vi "RunFileRenameAddDate.vi"() -> ()   [LabVIEW 2012]
panel:
  out "path out 3":path
  out "filenames 3":string[](array[string])
  out "folder names 3":string[](array[string])
  out "array":string[][](array[string])
  out "filenames":string[](array[string])
  out "folder names":string[](array[string])
  in  "path":path=path "G:/DCIM"
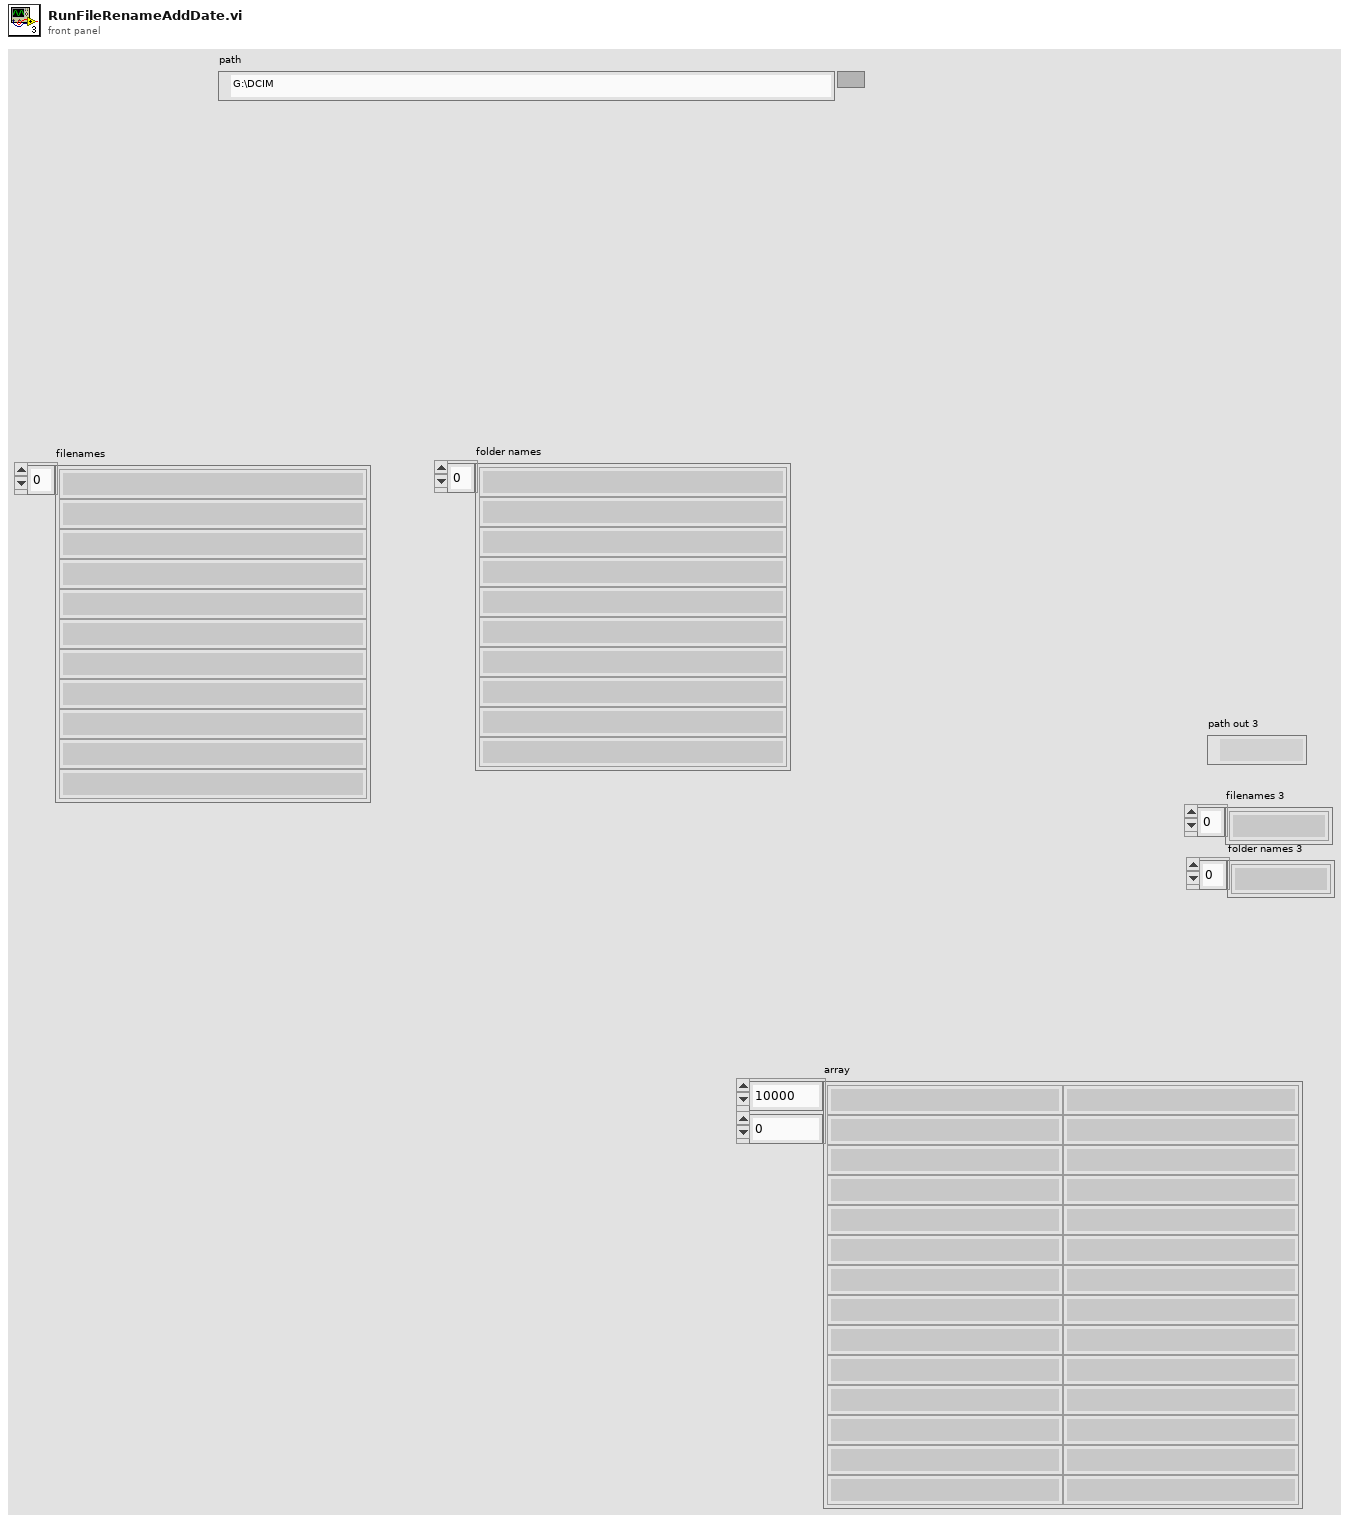
[diagram p1: front panel]
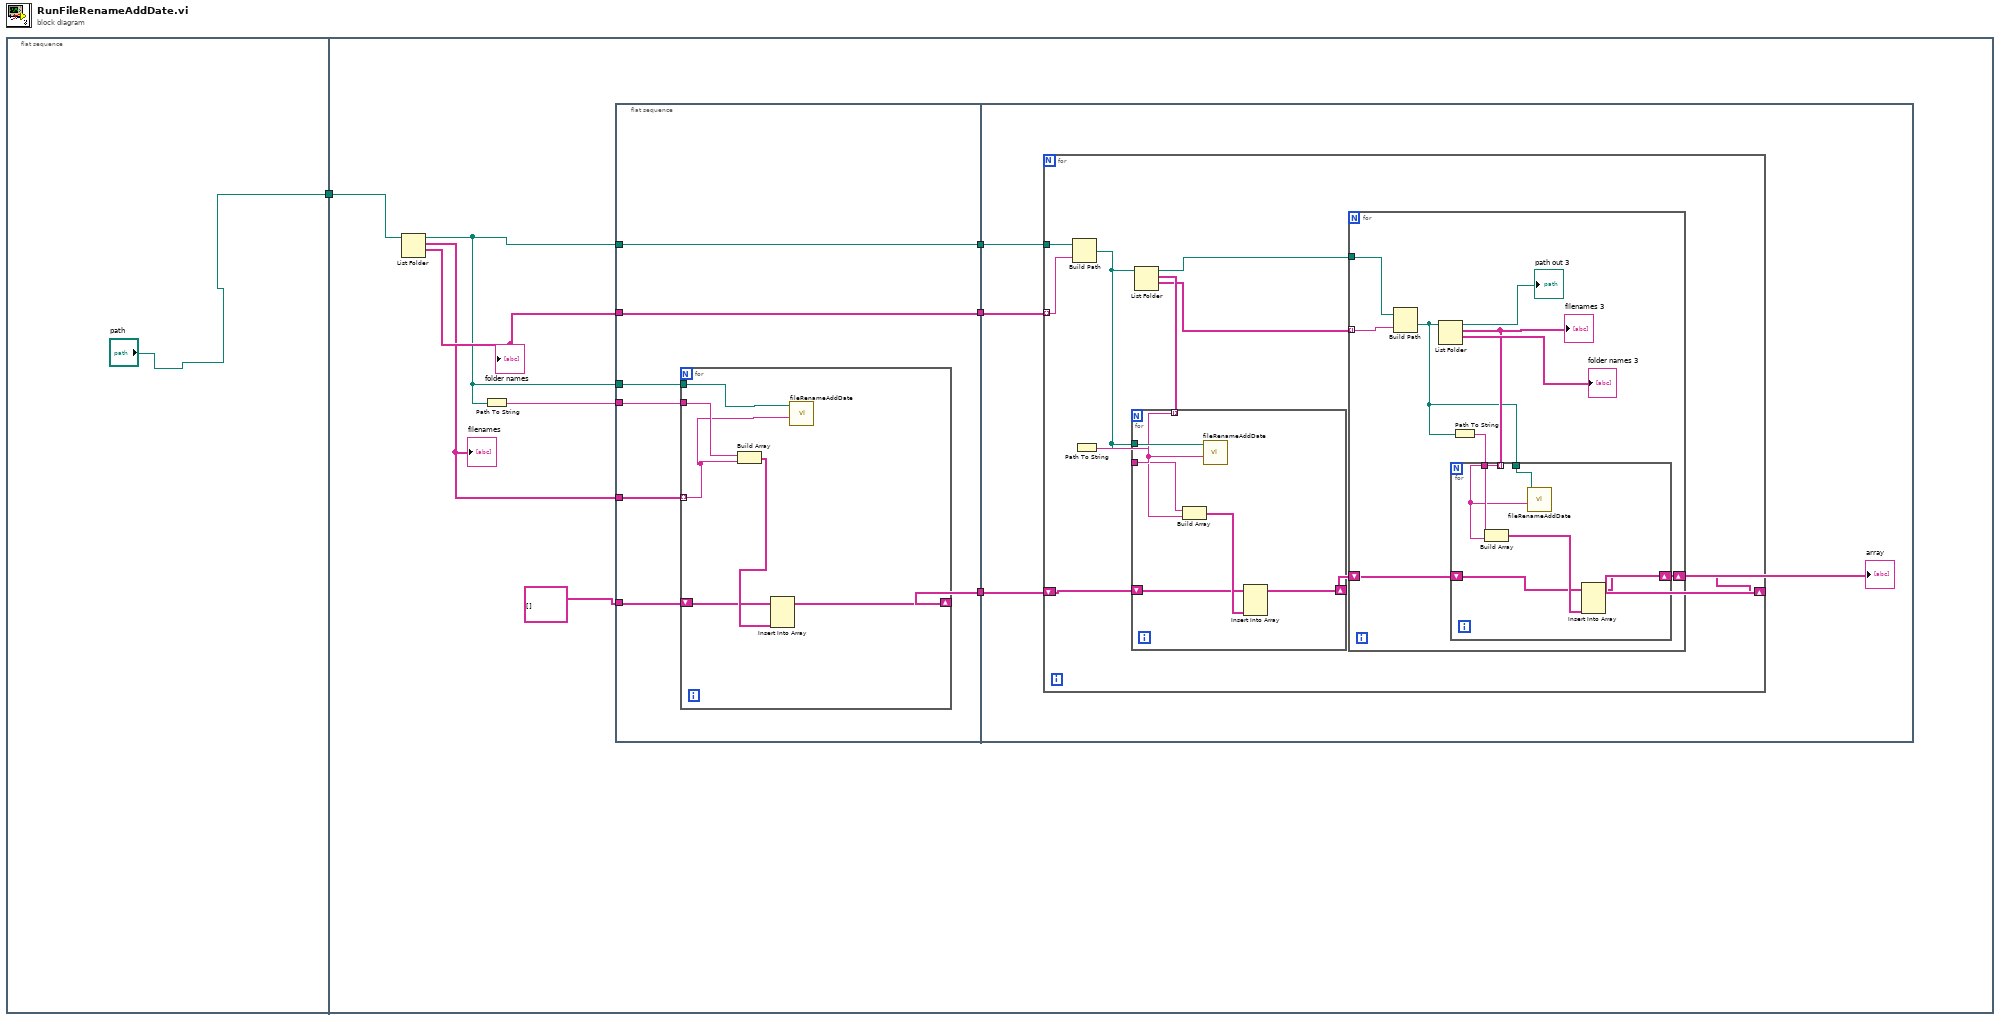
[diagram p0: block diagram]
diagram:
  n1 = flat-sequence {
    tunnel: ["path"] -> w1
    tunnel: w1 -> [w8]
    frame #0 {
    }
    frame #1 {
      n2 = List Folder(path=w8) -> (path out=w3:path, filenames=w4:string[], folder names=w7:string[])  [unwired: 3 in, 1 out]
      "filenames" <- w4
      "folder names" <- w7
      n3 = Path To String(path=w3) -> (string=w6:string)
      n4 = flat-sequence {
        tunnel: w3 -> [w17]
        tunnel: w7 -> [w18]
        tunnel: [w18] -> w11
        tunnel: [w17] -> w10
        tunnel: w4 -> [w16]
        tunnel: w6 -> [w15]
        tunnel: string[][] [] ("array") -> [w14]
        tunnel: [w13] -> w9
        tunnel: w3 -> [w12]
        tunnel: w11 -> [w28]
        tunnel: w10 -> [w27]
        tunnel: w9 -> [w26]
        frame #0 {
          n5 = for {
            tunnel: w16 -> [w19] mode=indexing
            tunnel: w15 -> [w24]
            shift-right: [w21] -> w13
            shift-left: w14 -> [w22]
            tunnel: w12 -> [w20]
            n6 = Build Array(w24, w19) -> (w23:string[])
            n7 = Insert Into Array(array=w22, new element=w23) -> (w21:string[][])  [unwired: 2 in]
            n8 = call "fileRenameAddDate.vi"("name or relative path"=w19, "base path"=w20) -> ()  [unwired: 10 in]
          }
        }
        frame #1 {
          n9 = for {
            tunnel: w28 -> [w38] mode=indexing
            tunnel: w27 -> [w37]
            shift-right: [w32] -> w25
            shift-left: w26 -> [w30]
            n10 = Build Path(base path=w37, name or relative path=w38) -> (appended path=w29:path)
            n11 = Path To String(path=w29) -> (string=w36:string)
            n12 = List Folder(path=w29) -> (path out=w34:path, filenames=w35:string[], folder names=w33:string[])  [unwired: 3 in, 1 out]
            n13 = for {
              tunnel: w36 -> [w44]
              tunnel: w35 -> [w39] mode=indexing
              shift-right: [w42] -> w31
              shift-left: w30 -> [w41]
              tunnel: w29 -> [w40]
              n14 = Build Array(w44, w39) -> (w43:string[])
              n15 = call "fileRenameAddDate.vi"("name or relative path"=w39, "base path"=w40) -> ()  [unwired: 10 in]
              n16 = Insert Into Array(array=w41, new element=w43) -> (w42:string[][])  [unwired: 2 in]
            }
            n17 = for {
              tunnel: w34 -> [w53]
              tunnel: w33 -> [w52] mode=indexing
              shift-right: [w48] -> w32
              shift-left: w31 -> [w46]
              n18 = Build Path(base path=w53, name or relative path=w52) -> (appended path=w45:path)
              n19 = List Folder(path=w45) -> (path out=→"path out 3":path, filenames=w47:string[], folder names=→"folder names 3":string[])  [unwired: 3 in, 1 out]
              "filenames 3" <- w47
              n20 = Path To String(path=w45) -> (string=w49:string)
              n21 = for {
                tunnel: w49 -> [w59]
                tunnel: w47 -> [w54] mode=indexing
                shift-right: [w57] -> w48
                shift-left: w46 -> [w56]
                tunnel: w45 -> [w55]
                n22 = Build Array(w59, w54) -> (w58:string[])
                n23 = call "fileRenameAddDate.vi"("name or relative path"=w54, "base path"=w55) -> ()  [unwired: 10 in]
                n24 = Insert Into Array(array=w56, new element=w58) -> (w57:string[][])  [unwired: 2 in]
              }
            }
          }
          "array" <- w25
        }
      }
    }
  }
